vi "Read Mod Infos.vi"(8 "error in (no error)":errorcluster, 11 "Chassis BOM in":refnum<class "Chassis BOM.lvclass">) -> (0 "error out":errorcluster, 2 "Mod Infos":T1[](array[typedef]), 3 "Chassis BOM out":refnum<class "Chassis BOM.lvclass">)   [LabVIEW 2018, in "Configuration Grandmaster.lvlib" / "Chassis BOM.lvclass"]
uses:
  Chassis BOM.lvclass
  DAQmx Mod Info.ctl
  Chassis BOM.lvclass/Chassis BOM.ctl
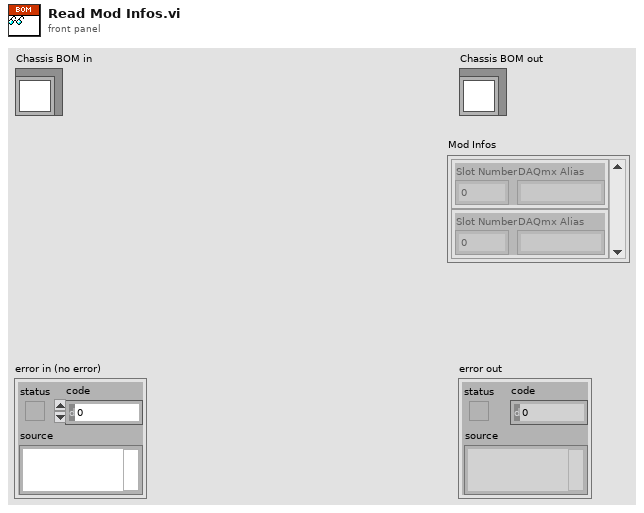
[diagram p1: front panel]
types:
  T1 = typedef "Configuration Grandmaster.lvlib/Chassis BOM.lvclass/DAQmx Mod Info.ctl" = cluster{"Slot Number":i32, "DAQmx Alias":string}
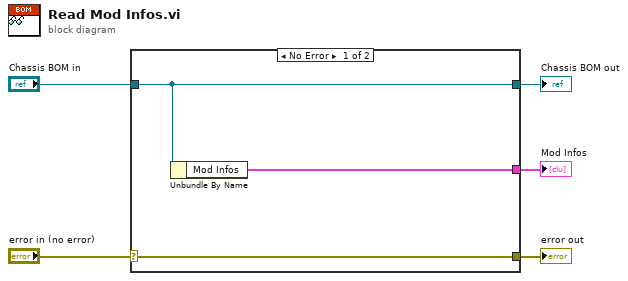
[diagram p0: block diagram]
diagram:
  n1 = case shown="No Error" "error in (no error)" {
    selector: "error in (no error)" -> [w8 w9]
    tunnel: [w8 w9] -> w4
    tunnel: [w7 w10] -> w2
    tunnel: "Chassis BOM in" -> [w7 w10]
    tunnel: [w6 _] -> w1
    frame No Error {
      n2 = Unbundle By Name(w7) -> ("Mod Infos"=w6:T1[])
    }
    frame Error {
    }
  }
  "error out" <- w4
  "Chassis BOM out" <- w2
  "Mod Infos" <- w1
